vi "xijk_save_to_file.vi"(8 "error in":errorcluster, 11 "save cluster":T1={{"axes in"={"min x-axis excitation"=0, "max x-axis excitation"=0, "min x-axis emission"=0, "max x-axis emission"=0, "precision of results"=2}, "plot colors in"={"Lanscape Portrait"=FALSE, "Plot logarithmic"=FALSE, "Ex/Em filters double"=FALSE, "Line colors"=[]}}, "search paths in"={"Paths"={"Path: Excitation filters"=path "", "Path: Dicroic filters"=path "", "Path: Emission filters"=path "", "Path reget"=path ""}, "table excitation"=[], "table dicroics"=[], "table emission"=[], "Integers"={"Select result n°"=0}, "boolean selector array"=[], "table for calculation automagic"=[]}, "spectra parameters in"={"Booleans"={"Notch filtering"=FALSE, "Unknown detector"=FALSE, "Dual band filters"=FALSE, "Dual emission by cubes"=FALSE, "FRET"=FALSE}, "Integers"={"Light source"=0, "Number of fluorophores"=0, "Wavelength of laser (nm) 1"=0, "Broadness of laser (nm) 1"=0, "Wavelength of laser (nm) 2"=0, "Broadness of laser (nm) 2"=0, "Template"=0}, "Doubles"={"Molar extinction 1"=0.0, "Molar extinction 2"=0.0, "Quantum efficiency 1"=0.0, "Quantum efficiency 2"=0.0}}, "filepaths in"={"Excitation filter 1"=path "", "Dichroic filter 1"=path "", "Emission filter 1"=path "", "Excitation filter 2"=path "", "Dichroic filter 2"=path "", "Emission filter 2"=path "", "Extra em filter 1"=path "", "Extra em filter 2"=path "", "Light source file"=path "", "Fluorophore absorption 1"=path "", "Fluorophore emission 1"=path "", "Fluorophore absorption 2"=path "", "Fluorophore emission 2"=path "", "Detector"=path ""}} {"?"."axes in"."precision of results" max=8 step=1}) -> (0 "error out":errorcluster)   [LabVIEW 2010]
uses:
  revised version/Type Def/save_cluster.ctl
  Type Def/axis_parameters.ctl
  revised version/Type Def/color_parameters.ctl
  Type Def/search_parameters.ctl
  Type Def/spectra_parameters.ctl
  Type Def/filepath.ctl
  <vilib>/Utility/xml.llb/Write to XML File(string).vi
panel:
  # "Dichroic"
  # "Ex/Em filter"
  # "Fluorophore 1"
  # "Fluorophore 2"
  # "Laser /\nextra Em filter"
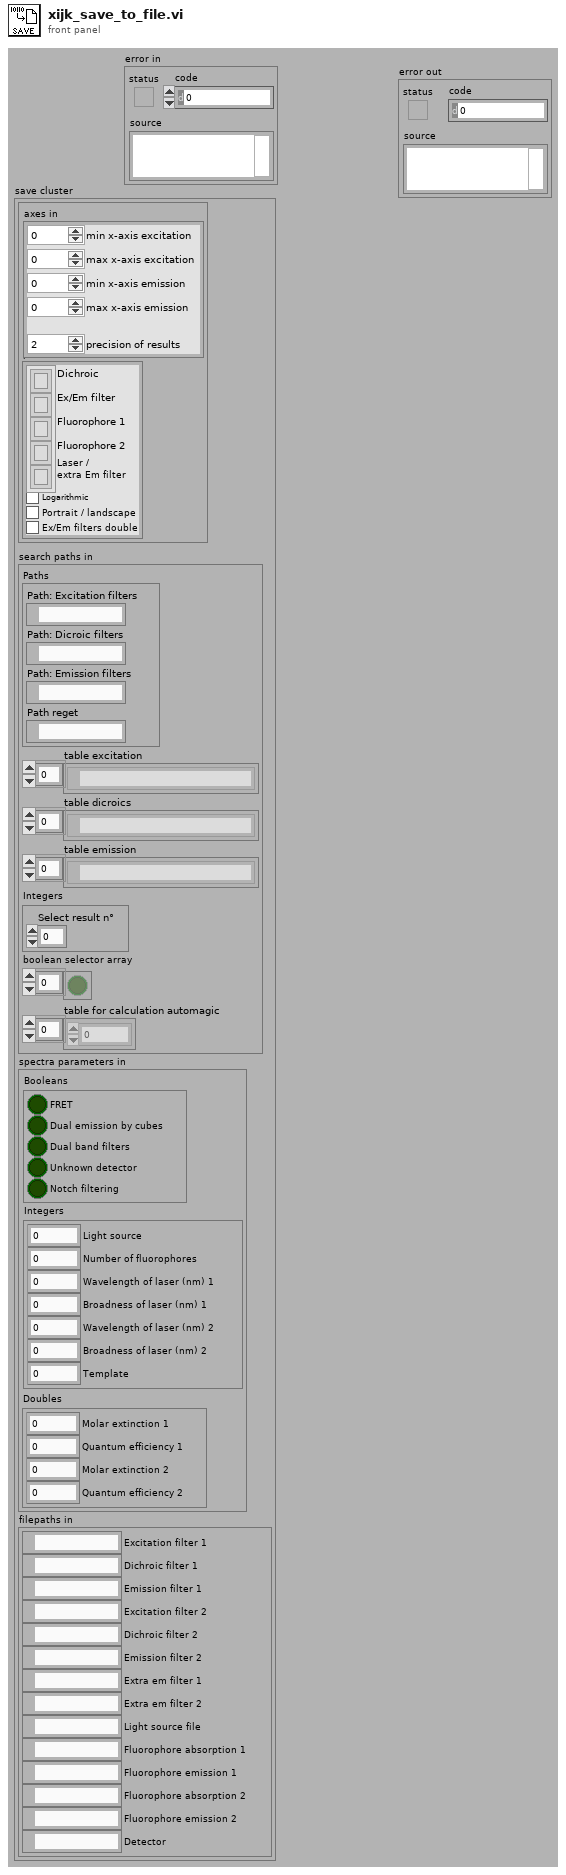
[diagram p1: front panel]
types:
  T1 = typedef "save_cluster.ctl" = cluster{cluster{"axes in":T2, "plot colors in":T3}, "search paths in":T4, "spectra parameters in":T5, "filepaths in":T6}
  T2 = typedef "axis_parameters.ctl" = cluster{"min x-axis excitation":u16, "max x-axis excitation":u16, "min x-axis emission":u16, "max x-axis emission":u16, "precision of results":u8}
  T3 = typedef "color_parameters.ctl" = cluster{"Lanscape Portrait":bool, "Plot logarithmic":bool, "Ex/Em filters double":bool, "Line colors":u32[]}
  T4 = typedef "search_parameters.ctl" = cluster{"Paths":cluster{"Path: Excitation filters":path, "Path: Dicroic filters":path, "Path: Emission filters":path, "Path reget":path}, "table excitation":path[], "table dicroics":path[], "table emission":path[], "Integers":cluster{"Select result n°":u32}, "boolean selector array":bool[], "table for calculation automagic":i32[]}
  T5 = typedef "spectra_parameters.ctl" = cluster{"Booleans":cluster{"Notch filtering":bool, "Unknown detector":bool, "Dual band filters":bool, "Dual emission by cubes":bool, "FRET":bool}, "Integers":cluster{"Light source":u16, "Number of fluorophores":u16, "Wavelength of laser (nm) 1":u16, "Broadness of laser (nm) 1":u16, "Wavelength of laser (nm) 2":u16, "Broadness of laser (nm) 2":u16, "Template":u16}, "Doubles":cluster{"Molar extinction 1":dbl, "Molar extinction 2":dbl, "Quantum efficiency 1":dbl, "Quantum efficiency 2":dbl}}
  T6 = typedef "filepath.ctl" = cluster{"Excitation filter 1":path, "Dichroic filter 1":path, "Emission filter 1":path, "Excitation filter 2":path, "Dichroic filter 2":path, "Emission filter 2":path, "Extra em filter 1":path, "Extra em filter 2":path, "Light source file":path, "Fluorophore absorption 1":path, "Fluorophore emission 1":path, "Fluorophore absorption 2":path, "Fluorophore emission 2":path, "Detector":path}
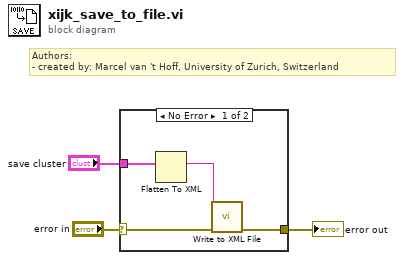
[diagram p0: block diagram]
diagram:
  # "Authors: \n- created by: Marcel van 't Hoff, University of Zurich, Switzerland"
  n1 = case shown="No Error" "error in" {
    selector: "error in" -> [w5 w8]
    tunnel: [w4 w8] -> w2
    tunnel: "save cluster" -> [w7 _]
    frame No Error {
      n2 = Flatten To XML(anything=w7) -> (xml string=w6:string)
      n3 = call-poly <vilib>:"Write to XML File.vi"("error in (no error)"=w5, "XML Input"=w6) -> ("error out"=w4:errorcluster)  [unwired: 7 in, 2 out]
    }
    frame Error {
    }
  }
  "error out" <- w2
